vi "1N.vi"(1 "Numeric":i32) -> (0 "Array":i32[](array[numeric]))   [LabVIEW 2018]
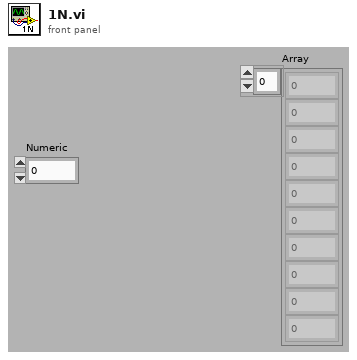
[diagram p1: front panel]
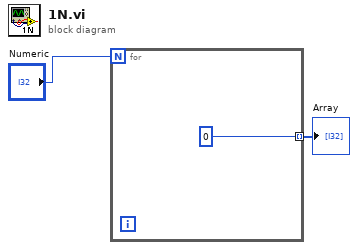
[diagram p0: block diagram]
diagram:
  n1 = for {
    N: "Numeric" -> [_]
    tunnel: [0] -> w1 mode=indexing
  }
  "Array" <- w1
